vi "Is a JKI State Machine.vi"(8 "error in (no error)":errorcluster, 11 "JKI SM in":refnum<class "JKI SM.lvclass">) -> (0 "error out":errorcluster, 2 "Is a JKI State Machine":bool, 3 "JKI SM out":refnum<class "JKI SM.lvclass">)   [LabVIEW 2013, in "JKI State Machine API.lvlib" / "JKI SM.lvclass"]
uses:
  JKI SM.lvclass
  JKI SM.lvclass/JKI SM.ctl
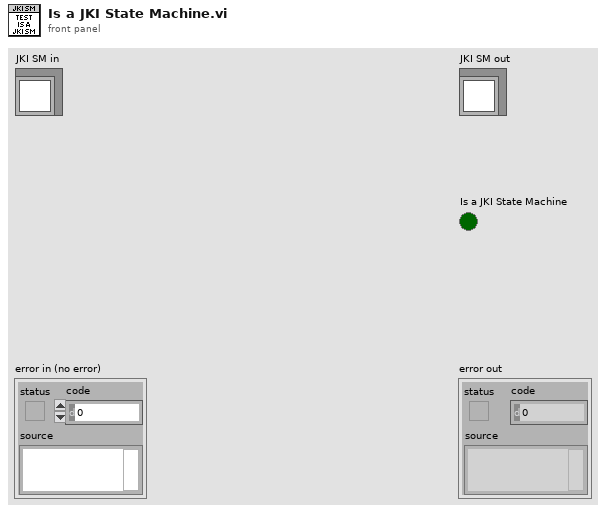
[diagram p1: front panel]
types:
  T1 = typedef "JKI State Machine API.lvlib/JKI SM.lvclass/Part References -- Cluster.ctl" = cluster{"While Loop":refnum<vi>, "Case Structure":refnum<vi>, "Event Structure":refnum<vi>, "Parse State Queue":refnum<vi>, "VI":refnum<vi>}
  T2 = cluster{"While Loop":bool, "Case Structure":bool, "Event Structure":bool, "Parse State Queue":bool, "VI":bool}
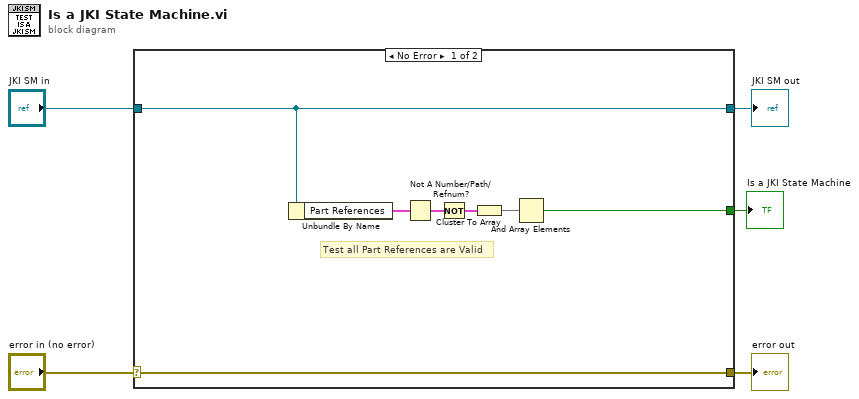
[diagram p0: block diagram]
diagram:
  n1 = case shown="No Error" "error in (no error)" {
    selector: "error in (no error)" -> [w12 w14]
    tunnel: [w12 w14] -> w4
    tunnel: [w11 w13] -> w2
    tunnel: "JKI SM in" -> [w11 w13]
    tunnel: [w7 _] -> w1
    frame No Error {
      # "Test all Part References are Valid"
      n2 = Unbundle By Name(w11) -> ("Part References"=w10:T1)
      n3 = Not A Number/Path/Refnum?(number/path/refnum=w10) -> (NaN/Path/Refnum?=w9:T2)
      n4 = Not(x=w9) -> (.not. x?=w6:T2)
      n5 = Cluster To Array(cluster=w6) -> (array=w8:bool[])
      n6 = And Array Elements(Boolean array=w8) -> (logical AND=w7:bool)
    }
    frame Error {
    }
  }
  "error out" <- w4
  "JKI SM out" <- w2
  "Is a JKI State Machine" <- w1
